vi "Pool.vi"(7 "Data":cluster{"Speed":dbl, "Angle":dbl, "Color":u32}) -> (0 "Simulation Objects":refnum<class "SimulationObject.lvclass">[](array[class]), 1 "Cell Size":i16, 2 "Gravity Vector out":refnum<class "Vector2.lvclass">, 3 "Background Color out":u32(colorbox))   [LabVIEW 2022 SP3]
uses:
  Engine/Math/Vector2/Vector2.lvclass
  Engine/Objects/SimulationObject/SimulationObject.lvclass
  Engine/Math/Vector2/Vector2.lvclass/Vector2.ctl
  Engine/Objects/SimulationObject/SimulationObject.lvclass/SimulationObject.ctl
  Engine/Objects/Components/PhysicsComponent/PhysicsComponent.lvclass/PhysicsComponent.ctl
  <vilib>/numeric/Random Number (Range) I64.vi
  <vilib>/numeric/sub_Random U32.vi
  Engine/Objects/Shapes/CircleShape/CircleShape.lvclass
  D:/Programowanie/Studia/Labview/CollisionSimulator/Project/Engine/Objects/Shapes/Shapeable/Shapeable.lvclass
  Engine/Objects/Components/PhysicsComponent/PhysicsComponent.lvclass
  D:/Programowanie/Studia/Labview/CollisionSimulator/Project/Engine/Objects/Shapes/CircleShape/CircleShape.lvclass
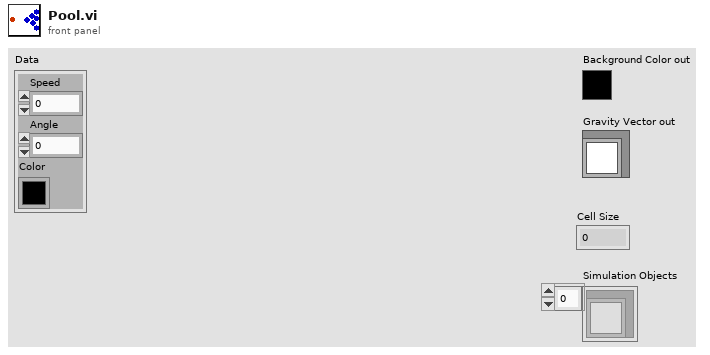
[diagram p1: front panel]
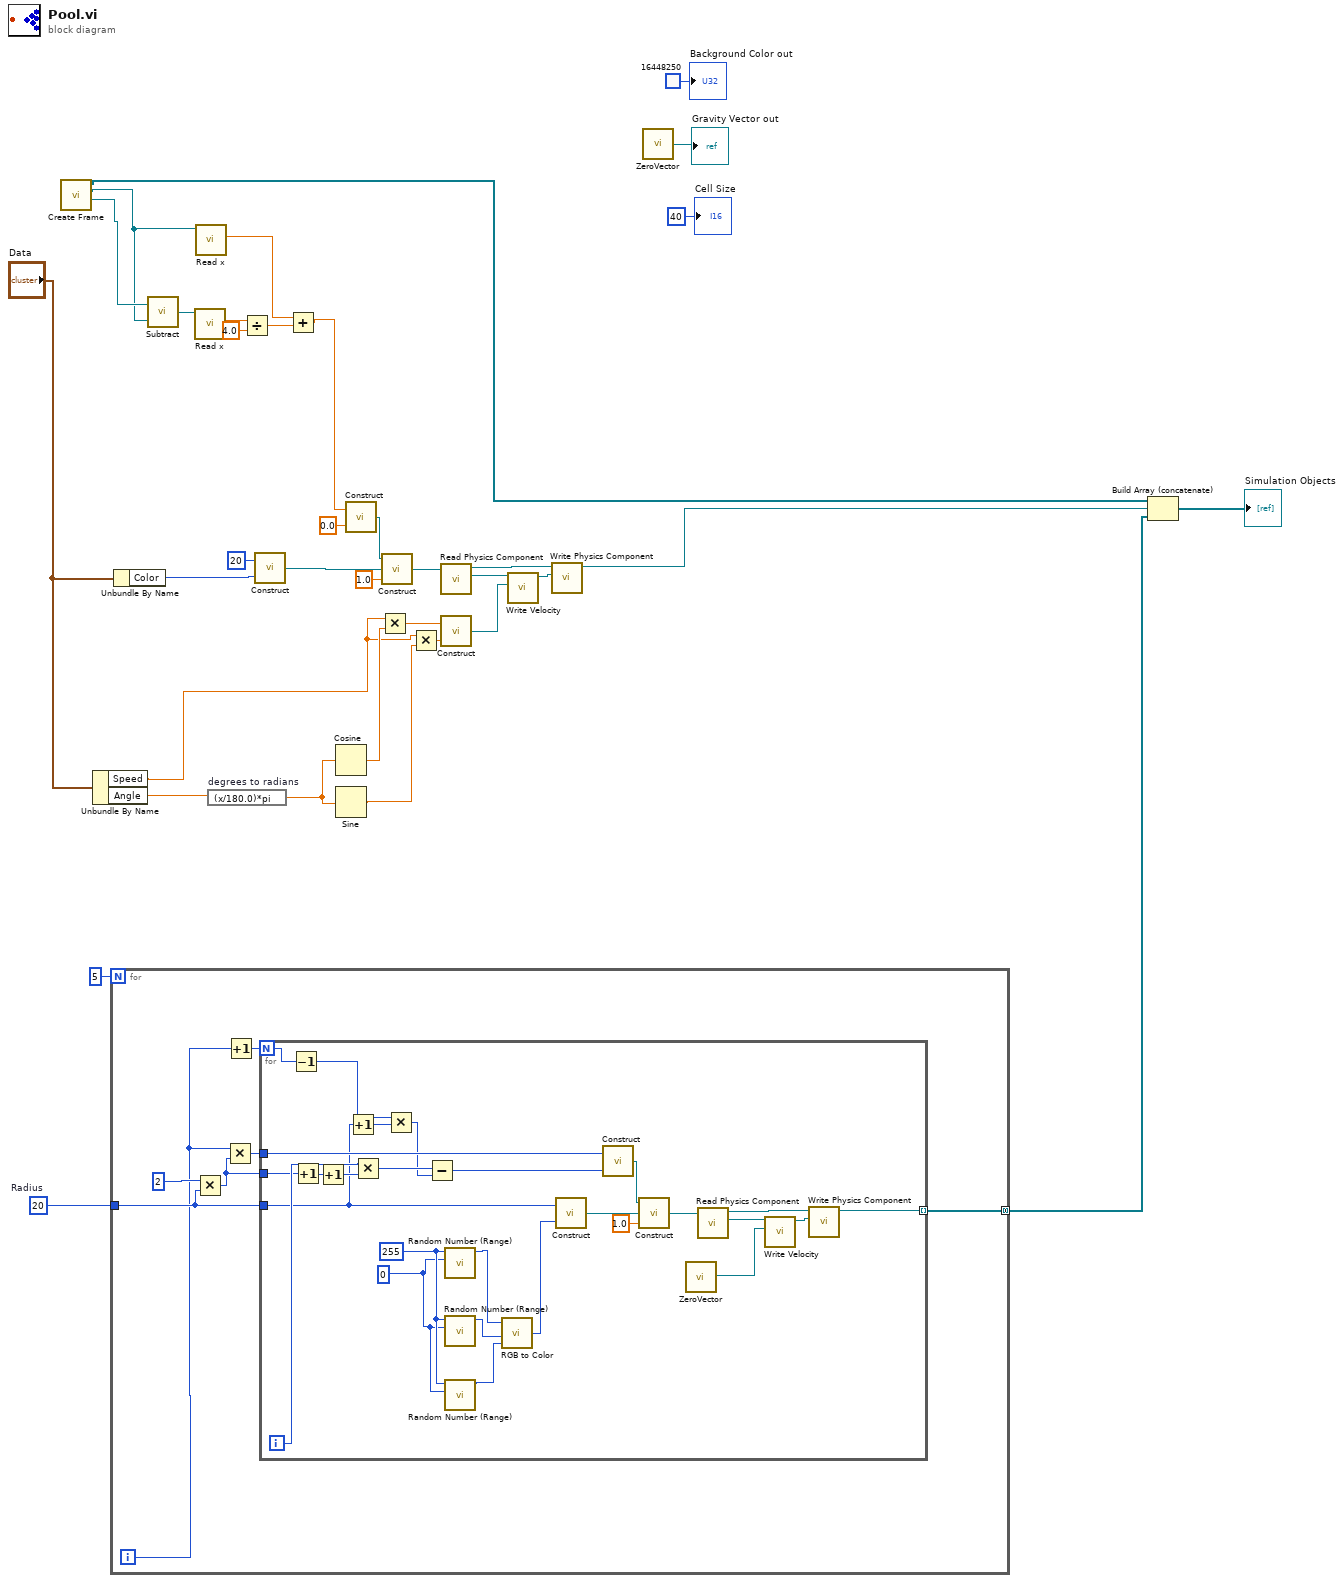
[diagram p0: block diagram]
diagram:
  w2 = i16 20  # Radius
  n1 = call "Create Frame.vi"() -> ("Max Available Position"=w9:refnum<class "Vector2.lvclass">, "Min Available Position"=w8:refnum<class "Vector2.lvclass">, "Simulation Objects"=w5:refnum<class "SimulationObject.lvclass">[])  [unwired: 4 in, 1 out]
  n2 = Unbundle By Name("Data") -> ("Speed"=w20:dbl, "Angle"=w21:dbl)
  n3 = for {
    N: 5 -> [_]
    tunnel: [w43] -> w1 mode=concatenating
    tunnel: w2 -> [w40]
    i -> [w37]
    n4 = Multiply(x=i16 2, y=w40) -> (x*y=w38:i16)
    n5 = Multiply(x=w37, y=w38) -> (x*y=w41:i32)
    n6 = Increment(x=w37) -> (x+1=w42:i32)
    n7 = for {
      N: w42 -> [w51]
      tunnel: [w56] -> w43 mode=indexing
      tunnel: w40 -> [w44]
      tunnel: w41 -> [w55]
      tunnel: w38 -> [w48]
      i -> [w54]
      w61 = 0
      w62 = 255
      n8 = Decrement(x=w51) -> (x-1=w50:i32)
      n9 = Increment(x=w48) -> (x+1=w47:i16)
      n10 = Increment(x=w47) -> (x+1=w46:i16)
      n11 = Increment(x=w44) -> (x+1=w45:i16)
      n12 = Multiply(x=w54, y=w46) -> (x*y=w53:i32)
      n13 = Multiply(x=w50, y=w45) -> (x*y=w49:i32)
      n14 = Subtract(x=w53, y=w49) -> (x-y=w52:i32)
      n15 = call-poly <vilib>:"Random Number (Range).vi"("lower bound (-100)"=w61, "upper bound (100)"=w62) -> ("number"=w59:i64)  [unwired: 9 in]
      n16 = call-poly <vilib>:"Random Number (Range).vi"("lower bound (-100)"=w61, "upper bound (100)"=w62) -> ("number"=w58:i64)  [unwired: 9 in]
      n17 = call-poly <vilib>:"Random Number (Range).vi"("lower bound (-100)"=w61, "upper bound (100)"=w62) -> ("number"=w57:i64)  [unwired: 9 in]
      n18 = call <vilib>:"RGB to Color.vi"("B"=w57, "G"=w58, "R"=w59) -> ("Color"=w60:u32)
      n19 = call "Construct.vi"("Color"=w60, "Radius"=w44) -> ("CircleShape out"=w70:refnum<class "CircleShape.lvclass">)
      n20 = call "Construct.vi"("y"=w52, "x"=w55) -> ("Vec2 out"=w69:refnum<class "Vector2.lvclass">)
      n21 = call "Construct.vi"("Mass"=sgl 1.0, "Shape in"=w70, "Local Position in"=w69) -> ("Simulation Object out"=w68:refnum<class "SimulationObject.lvclass">)
      n22 = call "ZeroVector.vi"() -> ("Zero Vector"=w63:refnum<class "Vector2.lvclass">)
      n23 = call "Read Physics Component.vi"("SimulationObject in"=w68) -> ("Physics Component out"=w65:refnum<class "PhysicsComponent.lvclass">, "SimulationObject out"=w67:refnum<class "SimulationObject.lvclass">)  [unwired: 8 in, 1 out]
      n24 = call "Write Velocity.vi"("Velocity in"=w63, "PhysicsComponent in"=w65) -> ("PhysicsComponent out"=w66:refnum<class "PhysicsComponent.lvclass">)  [unwired: 8 in, 1 out]
      n25 = call "Write Physics Component.vi"("PhysicsComponent.lvclass"=w66, "SimulationObject in"=w67) -> ("SimulationObject out"=w56:refnum<class "SimulationObject.lvclass">)  [unwired: 8 in, 1 out]
    }
  }
  n26 = Unbundle By Name("Data") -> ("Color"=w17:u32)
  n27 = call "Subtract.vi"("Vec2 b in"=w8, "Vec2 a in"=w9) -> ("Vec2 out"=w14:refnum<class "Vector2.lvclass">)
  n28 = call "Read x.vi"("Vector2 in"=w14) -> ("x"=w13:sgl)  [unwired: 8 in, 2 out]
  n29 = call "Read x.vi"("Vector2 in"=w8) -> ("x"=w11:sgl)  [unwired: 8 in, 2 out]
  n30 = expression code="(x/180.0)*pi" "degrees to radians"(w21) -> (w29:dbl)
  n31 = Divide(x=w13, y=sgl 4.0) -> (x/y=w10:sgl)
  n32 = call "Construct.vi"("Color"=w17, "Radius"=i16 20) -> ("CircleShape out"=w28:refnum<class "CircleShape.lvclass">)
  n33 = Add(x=w11, y=w10) -> (x+y=w7:sgl)
  n34 = Cosine(x=w29) -> (cos(x)=w32:dbl)
  n35 = Sine(x=w29) -> (sin(x)=w33:dbl)
  n36 = call "Construct.vi"("y"=sgl 0.0, "x"=w7) -> ("Vec2 out"=w27:refnum<class "Vector2.lvclass">)
  n37 = Multiply(x=w20, y=w32) -> (x*y=w30:dbl)
  n38 = call "Construct.vi"("Mass"=sgl 1.0, "Shape in"=w28, "Local Position in"=w27) -> ("Simulation Object out"=w26:refnum<class "SimulationObject.lvclass">)
  n39 = Multiply(x=w20, y=w33) -> (x*y=w31:dbl)
  n40 = call "Read Physics Component.vi"("SimulationObject in"=w26) -> ("Physics Component out"=w23:refnum<class "PhysicsComponent.lvclass">, "SimulationObject out"=w25:refnum<class "SimulationObject.lvclass">)  [unwired: 8 in, 1 out]
  n41 = call "Construct.vi"("y"=w31, "x"=w30) -> ("Vec2 out"=w22:refnum<class "Vector2.lvclass">)
  n42 = call "Write Velocity.vi"("Velocity in"=w22, "PhysicsComponent in"=w23) -> ("PhysicsComponent out"=w24:refnum<class "PhysicsComponent.lvclass">)  [unwired: 8 in, 1 out]
  n43 = call "Write Physics Component.vi"("PhysicsComponent.lvclass"=w24, "SimulationObject in"=w25) -> ("SimulationObject out"=w6:refnum<class "SimulationObject.lvclass">)  [unwired: 8 in, 1 out]
  n44 = call "ZeroVector.vi"() -> ("Zero Vector"=→"Gravity Vector out":refnum<class "Vector2.lvclass">)
  n45 = Build Array (concatenate)(w5, w6, w1) -> (→"Simulation Objects":refnum<class "SimulationObject.lvclass">[])
  "Background Color out" <- u32 16448250 ("Background Color out")
  "Cell Size" <- i16 40 ("Cell Size")
